vi "niFpgaFFTStreamingStages_256.vi"(0 "reset":bool, 1 "mult output type":fxp<+/-,18,2> format="%#.17g", 2 "bf bullet type":fxp<+,7,7>, 5 "bf data in":T1 {"x_r" format="%.16g"; "x_i" format="%.16g"; "y_r" format="%.16g"; "y_i" format="%.16g"}, 7 "stage switch in":bool, 9 "twiddle index in":fxp<+,6,6>, 11 "bf data type":T1 {"x_r" format="%.16g"; "x_i" format="%.16g"; "y_r" format="%.16g"; "y_i" format="%.16g"}) -> (6 "bf data out":T1 {"x_r" format="%.16g"; "x_i" format="%.16g"; "y_r" format="%.16g"; "y_i" format="%.16g"}, 8 "stage switch out":bool)   [LabVIEW 2017]
uses:
  <vilib>/rvi/Analysis/measure/FFT/supportingXNodes/permutation/templates/niFPGA FFT Perm Buffer 64 U32.vi
  <vilib>/rvi/Analysis/measure/FFT/supportingXNodes/BFGroup/templates/niFPGA BFGroup Input Buffer 256 U32.vi
  <vilib>/rvi/Analysis/measure/FFT/supportingXNodes/BFGroup/templates/niFPGA BFGroup Twiddle Table 128 U32.vi
  <vilib>/rvi/Analysis/measure/FFT/supportingXNodes/BFGroup/templates/niFPGA BFGroup Twiddle Table 32 U32.vi
  <vilib>/rvi/Analysis/measure/FFT/supportingXNodes/BFGroup/templates/niFPGA BFGroup Twiddle Table 8 U32.vi
  <vilib>/rvi/Analysis/measure/FFT/supportingXNodes/BFGroup/XNode/niFpgaFFTBFGroup.xnode
  <vilib>/rvi/FXPMathLib/basic elements/FxpDiscreteDelay/XNode/nifxpmath_DiscreteDelay.xnode
  <vilib>/rvi/Analysis/measure/FFT/supportingXNodes/permutation/XNode/niFpgaFFTPermutation.xnode
  <vilib>/rvi/Analysis/measure/FFT/supportingXNodes/butterfly/XNode/niFpgaFFTDIFButterfly.xnode
  <vilib>/rvi/FXPMathLib/FxpMul/XNode/nifxpmath_Multiplier.xnode
  <vilib>/rvi/FXPMathLib/sim/FxpSim.dll
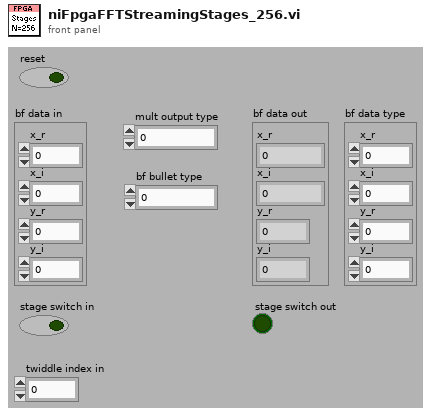
[diagram p1: front panel]
types:
  T1 = cluster{"x_r":fxp<+/-,16,1>, "x_i ":fxp<+/-,16,1>, "y_r ":fxp<+/-,16,1>, "y_i ":fxp<+/-,16,1>}
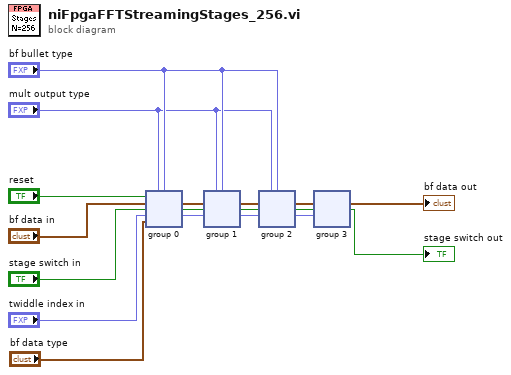
[diagram p0: block diagram]
diagram:
  n1 = xnode "group 0"("mult output type"="mult output type", "bf data in"="bf data in", "stage switch in"="stage switch in", "tf index in"="twiddle index in", "reset"="reset", "bf bullet type"="bf bullet type", "bf data type"="bf data type") -> ("stage switch out"=w15:bool, "bf data out"=w18:T1, "tf index out"=w12:fxp<+,7,7>)
  n2 = xnode "group 1"("mult output type"="mult output type", "bf data in"=w18, "stage switch in"=w15, "tf index in"=w12, "bf bullet type"="bf bullet type") -> ("stage switch out"=w14:bool, "bf data out"=w17:T1, "tf index out"=w11:fxp<+,7,7>)
  n3 = xnode "group 2"("mult output type"="mult output type", "bf data in"=w17, "stage switch in"=w14, "tf index in"=w11, "bf bullet type"="bf bullet type") -> ("stage switch out"=w13:bool, "bf data out"=w16:T1, "tf index out"=w10:fxp<+,7,7>)
  n4 = xnode "group 3"("bf data in"=w16, "stage switch in"=w13, "tf index in"=w10) -> ("stage switch out"=→"stage switch out":bool, "bf data out"=→"bf data out":T1)
